vi "Savitzky-Golay Filter Coefficients.vi"(8 "Weight":dbl[](array[numeric]), 9 "polynomial order":i32=3, 10 "side points":i32=6, 11 "compute differentiation filters?":bool=TRUE) -> (0 "error":i32, 2 "Differentiation Filters":T1, 3 "Savitzky-Golay Filters":T1)   [LabVIEW 2017, in "NI_AALBase.lvlib"]
doc: "Designs a Savitzky-Golay FIR smoothing filter. This VI returns the designed Savitzky-Golay filter coefficients and the differentiation filter coefficients."
uses:
  <vilib>/Analysis/NI_AALBase.lvlib
  <vilib>/Analysis/Matrix/Datatypes/RealMatrix.ctl
  <resource>/lvanlys.dll
  <vilib>/Analysis/Matrix/NI_Matrix.lvlib
panel:
  # "Savitzky-Golay Filter Coefficients"
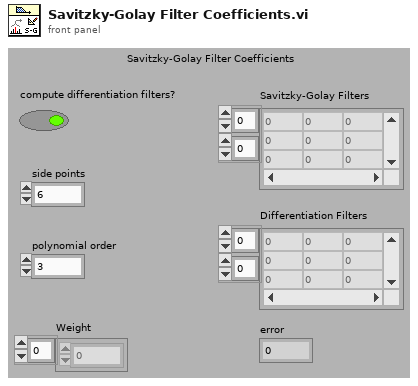
[diagram p1: front panel]
types:
  T1 = typedef "NI_Matrix.lvlib/RealMatrix.ctl" = dbl[][]
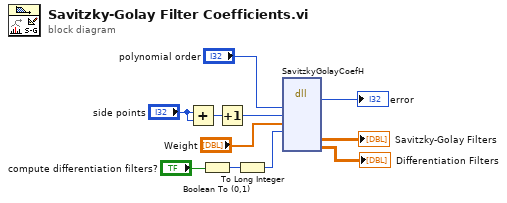
[diagram p0: block diagram]
diagram:
  n1 = Add(x="side points", y="side points") -> (x+y=w3:i32)
  n2 = Boolean To (0,1)(Boolean="compute differentiation filters?") -> (0, 1=w7:i16)
  n3 = Increment(x=w3) -> (x+1=w1:i32)
  n4 = To Long Integer(number=w7) -> (32bit integer=w6:i32)
  n5 = dll-call lib="e:/builds/penguin/labview/branches/2017/dev/dist/resource/lvanlys.*" fn="SavitzkyGolayCoefH"("polyOrder"="polynomial order", "frameSize"=w1, "weight"="Weight", "needDiff"=w6) -> (→"error":i32, "filterCoeffs"=→"Savitzky-Golay Filters":dbl[][], "diffCoefs"=→"Differentiation Filters":dbl[][])  [unwired: 9 in, 2 out]
